vi "FixPGCam.vi"(8 "error in":errorcluster, 11 "Session In":T1) -> (0 "error out":errorcluster, 3 "IMAQdx Session Out":T1)   [LabVIEW 2014]
uses:
  <vilib>/vision/driver/IMAQdx.llb/IMAQdx Attribute Type.ctl
  <vilib>/userdefined/High Color/IMAQdx.ctl
  <vilib>/vision/driver/NI_Vision_Acquisition_Software.lvlib
  <resource>/objmgr/imaqdx.rc
panel:
  out "Attribute Name":string
  out "Attribute Information Array":T3(array[cluster])
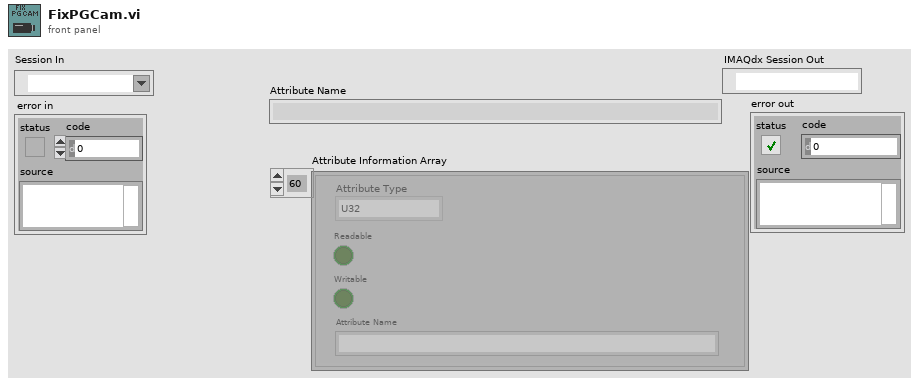
[diagram p1: front panel]
types:
  T1 = typedef "IMAQdx.ctl" = refnum<k21>
  T2 = typedef "NI_Vision_Acquisition_Software.lvlib/IMAQdx Attribute Type.ctl" = enum32{"U32", "I64", "DBL", "String", "Enum", "Bool", "Command"}
  T3 = cluster{"Attribute Type":T2, "Readable":bool, "Writable":bool, "Attribute Name":string}[]
  T4 = cluster{"Attribute Type":T2, "Readable":bool, "Writable":bool, "Attribute Name":string}
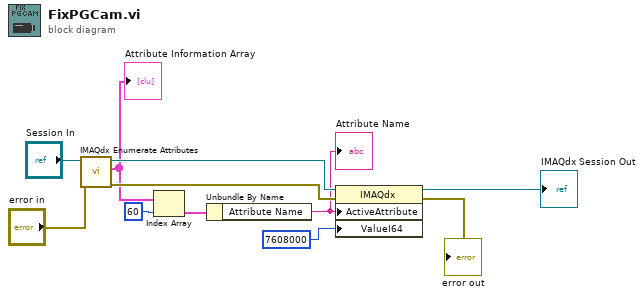
[diagram p0: block diagram]
diagram:
  n1 = call <vilib>:"IMAQdx Enumerate Attributes.vi"("error in"="error in", "Session In"="Session In") -> ("error out"=w11:errorcluster, "Attribute Information Array"=w9:T3, "Session Out"=w10:T1)  [unwired: 7 in]
  "Attribute Information Array" <- w9
  n2 = Index Array(array=w9, index=60) -> (element=w7:T4)
  n3 = Unbundle By Name(w7) -> ("Attribute Name"=w6:string)
  "Attribute Name" <- w6
  n4 = property class="IMAQdx"(reference=w10, error in=w11, "ActiveAttribute"=w6, "ValueI64"=i64 7608000) -> (reference out=→"IMAQdx Session Out":T1, error out=→"error out":errorcluster)
